vi "gfitsio-open-create-replace-file.vi"(4 "advisory dialog? (display:T)":bool=TRUE, 5 "prompt":string, 6 "default name":string, 8 "error in (no error)":errorcluster, 9 "function (open)":T2(ring), 11 "file path (dialog if empty)":path) -> (0 "error out":errorcluster, 2 "new file path":path, 3 "gfits refnum":T1)   [LabVIEW 2013, in "gfitsio.lvlib"]
doc: "Opens an existing FITS file, creates a new FITS file, or replaces an existing FITS file, programmatically or interactively using a file dialog box. You can optionally specify a dialog prompt and default file name."
uses:
  gfitsio.lvlib
  gfitsio-refnum.ctl
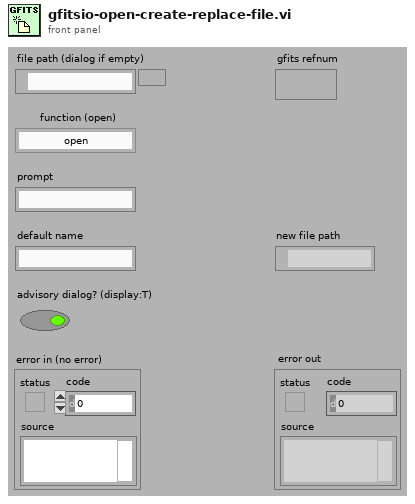
[diagram p1: front panel]
types:
  T1 = typedef "gfitsio.lvlib/gfitsio-refnum.ctl" = refnum<k1>
  T2 = enum16{"open", "open or create", "create or replace", "create", "open (read only)"}
  T3 = enum32{"existing file", "new file", "new or existing file", "existing dir", "new dir", "new or existing dir", "existing file (use LLBs)", "new file (use LLBs)", "new or existing file (use LLBs)", "new or existing file or directory (use LLBs)"}[]
  T4 = enum32{"existing file", "new file", "new or existing file", "existing dir", "new dir", "new or existing dir", "existing file (use LLBs)", "new file (use LLBs)", "new or existing file (use LLBs)", "new or existing file or directory (use LLBs)"}
  T5 = enum16{"Error", "Ok", "Cancel", "Abort", "Retry", "Ignore", "Yes", "No", "Close", "Help", "Disabled"}
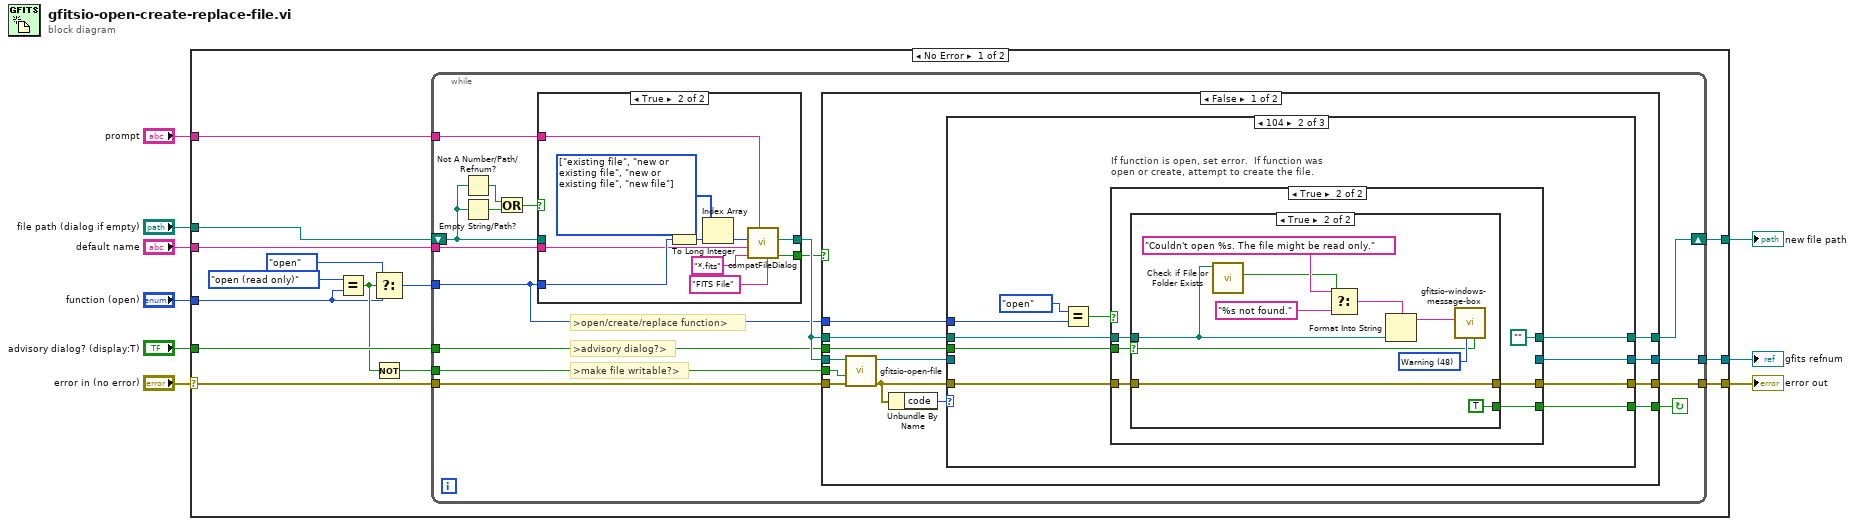
[diagram p0: block diagram]
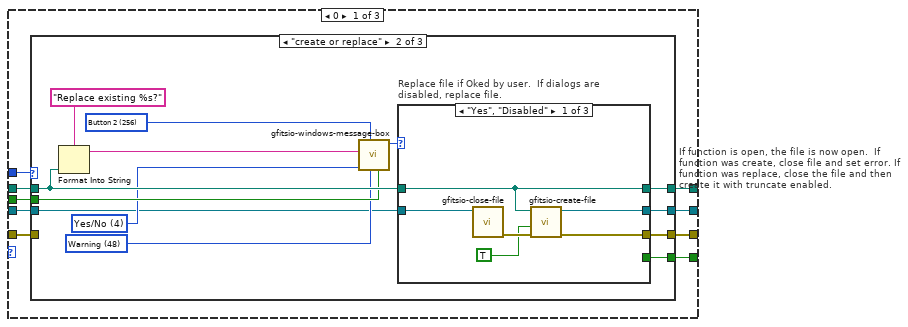
[diagram p3: hidden frame]
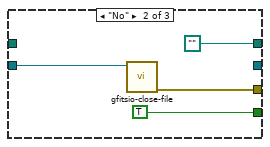
[diagram p5: hidden frame]
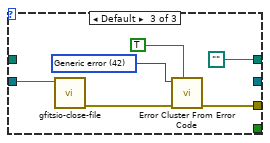
[diagram p6: hidden frame]
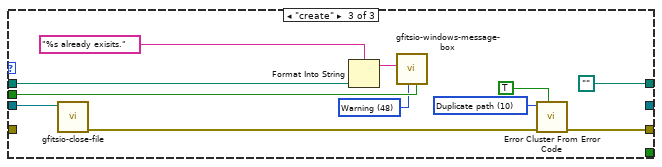
[diagram p7: hidden frame]
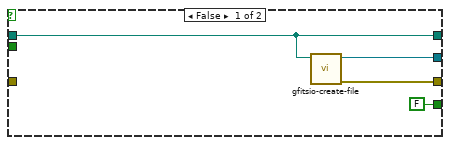
[diagram p8: hidden frame]
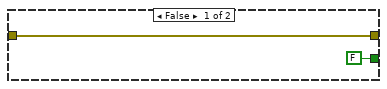
[diagram p9: hidden frame]
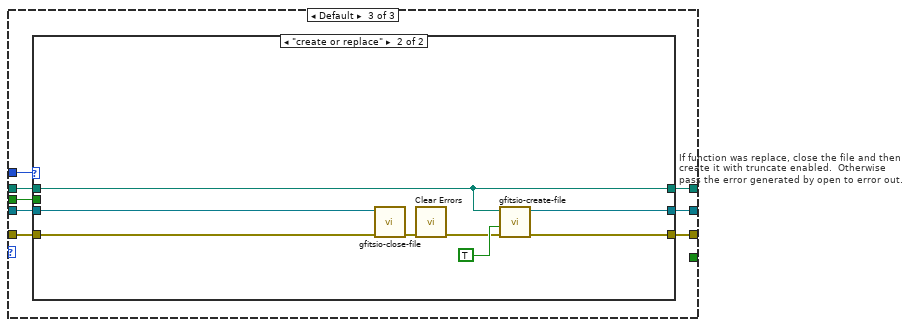
[diagram p10: hidden frame]
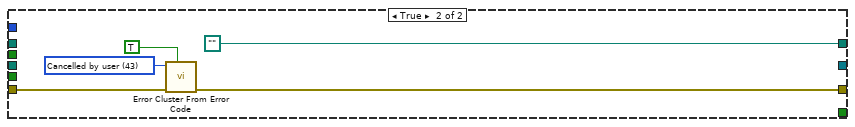
[diagram p12: hidden frame]
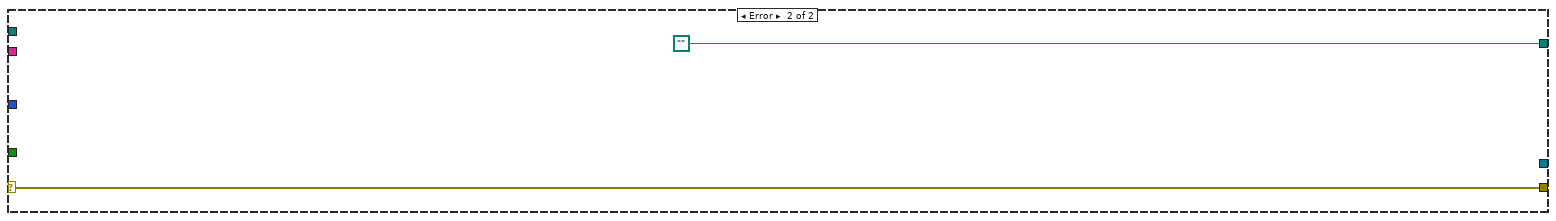
[diagram p13: hidden frame]
diagram:
  n1 = case shown="No Error" "error in (no error)" {
    selector: "error in (no error)" -> [w20 w172]
    tunnel: [w23 w172] -> w9
    tunnel: "advisory dialog? (display:T)" -> [w22 _]
    tunnel: [w21 path ""] -> w8
    tunnel: "default name" -> [w19 _]
    tunnel: "file path (dialog if empty)" -> [w18 _]
    tunnel: "prompt" -> [w17 _]
    tunnel: [w16 _] -> w3
    tunnel: "function (open)" -> [w11 _]
    frame No Error {
      n2 = Equal?(x=T2."open (read only)" ("y"), y=w11) -> (x = y?=w15:bool)
      n3 = Select(t=T2."open", s=w15, f=w11) -> (s? t:f=w12:T2)
      n4 = Not(x=w15) -> (.not. x?=w10:bool)
      n5 = while {
        tunnel: [w39] -> w23
        tunnel: w22 -> [w34]
        tunnel: w20 -> [w32]
        tunnel: w12 -> [w31]
        tunnel: w19 -> [w29]
        tunnel: w17 -> [w27]
        tunnel: w10 -> [w25]
        tunnel: [w24] -> w16
        shift-right: [w33] -> w21
        shift-left: w18 -> [w28]
        stop <- w26 continue-if-true
        # ">open/create/replace function>"
        # ">make file writable?>"
        # ">advisory dialog?>"
        n6 = Not A Number/Path/Refnum?(number/path/refnum=w28) -> (NaN/Path/Refnum?=w37:bool)
        n7 = Empty String/Path?(string/path=w28) -> (empty?=w36:bool)
        n8 = Or(x=w37, y=w36) -> (x .or. y?=w38:bool)
        n9 = case shown="True" w38 {
          tunnel: [_ w50] -> w30
          tunnel: [w40 w49] -> w35
          tunnel: w31 -> [_ w48]
          tunnel: w27 -> [_ w45]
          tunnel: w29 -> [_ w44]
          tunnel: w28 -> [w40 _]
          frame False {
            # "a File Path is supplied (not empty); proceed"
          }
          frame True {
            w46 = T3 [enum."existing file", enum."new or existing file", enum."new or existing file", enum."new file"] items=["existing file", "new file", "new or existing file", "existing dir", "new dir", "new or existing dir", "existing file (use LLBs)", "new file (use LLBs)", "new or existing file (use LLBs)", "new or existing file or directory (use LLBs)"]
            n10 = To Long Integer(number=w48) -> (32bit integer=w41:i32)
            n11 = Index Array(array=w46, index=w41) -> (element=w47:T4)
            n12 = call <vilib>:"compatFileDialog.vi"("pattern label"="FITS File", "prompt"=w45, "pattern"="*.fits", "default name"=w44, "select mode (2)"=w47) -> ("cancelled"=w50:bool, "path"=w49:path)  [unwired: 2 in, 3 out]
          }
        }
        n13 = case shown="False" w30 {
          tunnel: w31 -> [w63 _]
          tunnel: w32 -> [w62 w169]
          tunnel: [w58 w168] -> w39
          tunnel: w35 -> [w61 _]
          tunnel: w35 -> [w60 _]
          tunnel: w34 -> [w59 _]
          tunnel: [w57 path ""] -> w33
          tunnel: [w54 _] -> w26
          tunnel: w25 -> [w53 _]
          tunnel: [w51 _] -> w24
          frame False {
            n14 = call "gfitsio-open-file.vi"("error in (no error)"=w62, "read only? (T:no)"=w53, "path"=w61) -> ("error out"=w55:errorcluster, "gfits refnum"=w52:T1)  [unwired: 7 out]
            n15 = Unbundle By Name(w55) -> ("code"=w56:i32)
            n16 = case shown="104" w56 {
              tunnel: w63 -> [w72 w124 w155]
              tunnel: w60 -> [w70 w123 w153]
              tunnel: w59 -> [w71 w122 w154]
              tunnel: [w68 w121 w151] -> w58
              tunnel: [w69 w120 w152] -> w57
              tunnel: w55 -> [w67 w118 w150]
              tunnel: [w66 w116 _] -> w54
              tunnel: w52 -> [w65 _ w148]
              tunnel: [w64 w117 w149] -> w51
              frame 0 {
                n17 = case "If function is open, the file is now open.  If function was create, close file and set error. If function was replace, close the file and then create it with truncate enabled." shown="\"create or replace\"" w72 {
                  tunnel: w71 -> [_ w85 w114]
                  tunnel: w70 -> [w75 w86 w113]
                  tunnel: [w75 w88 path ""] -> w69
                  tunnel: w67 -> [w74 _ _]
                  tunnel: [w74 w87 w111] -> w68
                  tunnel: [_ w79 _] -> w66
                  tunnel: w65 -> [w73 w77 w105]
                  tunnel: [w73 w76 _] -> w64
                  frame "open", "open or create", "open (read only)" {
                  }
                  frame "create or replace" {
                    w80 = u32 256 items=["Button 1"=0, "Button 2"=256, "Button 3"=512, "Button 4"=1024] ("Default (Button 1)")
                    w81 = u32 4 items=["Abort/Retry/Ignore"=2, "OK"=0, "OK/Cancel"=1, "Retry/Cancel"=5, "Yes/No"=4, "Yes/No/Cancel"=3] ("Buttons (OK)")
                    w82 = u32 48 items=["None"=0, "Warning"=48, "Confirmation"=64, "Question"=32, "Error"=16, "User Icon"=128] ("Icon (None)")
                    n18 = Format Into String(format string="Replace existing %s?", w86) -> (resulting string=w78:string)  [unwired: 2 in, 1 out]
                    n19 = call "gfitsio-windows-message-box.vi"("enable dialog?"=w85, "Icon (None)"=w82, "Default (Button 1)"=w80, "Buttons (OK)"=w81, "Text"=w78) -> ("Button Selected"=w83:T5)  [unwired: 3 in, 3 out]
                    n20 = case "Replace file if Oked by user.  If dialogs are disabled, replace file." shown="\"Yes\", \"Disabled\"" w83 {
                      tunnel: [w92 path "" path ""] -> w88
                      tunnel: [w93 w97 w102] -> w87
                      tunnel: w86 -> [w92 _ _]
                      tunnel: [_ TRUE _] -> w79
                      tunnel: w77 -> [w90 w95 w99]
                      tunnel: [w89 _ _] -> w76
                      frame "Yes", "Disabled" {
                        n21 = call "gfitsio-close-file.vi"("gfits refnum"=w90) -> ("error out"=w94:errorcluster)  [unwired: 1 in, 9 out]
                        n22 = call "gfitsio-create-file.vi"("error in (no error)"=w94, "overwrite? (F:no)"=TRUE ("overwrite (F)"), "path"=w92) -> ("error out"=w93:errorcluster, "gfits refnum"=w89:T1)  [unwired: 7 out]
                      }
                      frame "No" {
                        n23 = call "gfitsio-close-file.vi"("gfits refnum"=w95) -> ("error out"=w97:errorcluster)  [unwired: 1 in, 9 out]
                      }
                      frame Default {
                        w101 = 42 items=["No error", "Argument error", "Memory is full", "Out of zone", "End of file", "File already open", "Generic file I/O error", "File not found", "File permission error", "Disk is full", "Duplicate path", "Too many files open", "System feature not enabled", "Resource file not found", "Cannot add resource", "Resource not found", "Image not found", "Image memory error", "Pen does not exist", "Config type invalid", "Config token not found", "Config parse error", "Config memory error", "Bad external code format", "Bad external code offset", "External code not present", "Null window", "Destroy window error", "Null menu", "Print aborted", "Bad print record", "Print driver error", "Windows error during printing", "Memory error during printing", "Print dialog error", "Generic print error", "Invalid device refnum", "Device not found", "Device parameter error", "Device unit error", "Cannot open device", "Device call aborted", "Generic error", "Cancelled by user", "Object ID too low", "Object ID too high", "Object not in heap", "Unknown heap", "Unknown object (invalid DefProc)", "Unknown object (DefProc not in table)", "Message out of range", "Invalid (null) method", "Unknown message", "Manager call not supported", "Bad address", "Network operation in progress", "Network operation timed out", "Connection is busy", "Network attribute not supported", "Network error", "Address in use", "System out of memory", "Connection aborted", "Connection refused", "Not connected", "Already connected", "Connection closed", "Initialization error (interapplication manager)", "Bad occurrence", "Wait on unbound occurrence handler", "Occurrence queue overflow", "Datalog type conflict", "Unused", "Unrecognized type (interapplication manager)", "Memory corrupt", "Failed to make temporary DLL", "Old CIN version", "Drag socket not found", "Failed to load drop-object", "Failed to register OLE object", "Failed to release OLE object", "Format specifier type mismatch", "Unknown format specifier", "Too few format specifiers", "Too many format specifiers", "Scan failed", "Newer CIN version", "Error converting to variant", "Runtime menu error", "Password tampered", "Variant attribute not found", "Incompatible variant data type", "Event data is not available", "Event Store is not present", "Occurrence is not found", "Event Queue is not created", "Event info is not available in the type library", "Refnum passed is NULL", "Error retrieving Class GUID", "Error retrieving CoClass GUID", "Error retrieving TypeLib GUID.", "Bad built application magic bytes.", "Specific driver is different from the specific driver associated with the Logical Name.", "There is no session opened to the class driver.", "Max Error", "MAX - Error with config objects", "MAX - Error loading configuration", "MAX - Group not supported", "Singlecast connections can not send to multicast addresses.", "Multicast connections can not send to singlecast addresses.", "Specified IP address not in multicast address range.", "Attempt to write to read-only multicast connection.", "Attempt to read from write-only multicast connection.", "The buffer used to receive a datagram was smaller than the datagram itself"]
                        n24 = call "gfitsio-close-file.vi"("gfits refnum"=w99) -> ("error out"=w103:errorcluster)  [unwired: 1 in, 9 out]
                        n25 = call <vilib>:"Error Cluster From Error Code.vi"("show call chain? (False)"=TRUE, "error in (no error)"=w103, "error code (0)"=w101) -> ("error out"=w102:errorcluster)  [unwired: 6 out]
                      }
                    }
                  }
                  frame "create" {
                    w106 = u32 48 items=["None"=0, "Warning"=48, "Confirmation"=64, "Question"=32, "Error"=16, "User Icon"=128] ("Icon (None)")
                    w109 = 10 items=["No error", "Argument error", "Memory is full", "Out of zone", "End of file", "File already open", "Generic file I/O error", "File not found", "File permission error", "Disk is full", "Duplicate path", "Too many files open", "System feature not enabled", "Resource file not found", "Cannot add resource", "Resource not found", "Image not found", "Image memory error", "Pen does not exist", "Config type invalid", "Config token not found", "Config parse error", "Config memory error", "Bad external code format", "Bad external code offset", "External code not present", "Null window", "Destroy window error", "Null menu", "Print aborted", "Bad print record", "Print driver error", "Windows error during printing", "Memory error during printing", "Print dialog error", "Generic print error", "Invalid device refnum", "Device not found", "Device parameter error", "Device unit error", "Cannot open device", "Device call aborted", "Generic error", "Cancelled by user", "Object ID too low", "Object ID too high", "Object not in heap", "Unknown heap", "Unknown object (invalid DefProc)", "Unknown object (DefProc not in table)", "Message out of range", "Invalid (null) method", "Unknown message", "Manager call not supported", "Bad address", "Network operation in progress", "Network operation timed out", "Connection is busy", "Network attribute not supported", "Network error", "Address in use", "System out of memory", "Connection aborted", "Connection refused", "Not connected", "Already connected", "Connection closed", "Initialization error (interapplication manager)", "Bad occurrence", "Wait on unbound occurrence handler", "Occurrence queue overflow", "Datalog type conflict", "Unused", "Unrecognized type (interapplication manager)", "Memory corrupt", "Failed to make temporary DLL", "Old CIN version", "Drag socket not found", "Failed to load drop-object", "Failed to register OLE object", "Failed to release OLE object", "Format specifier type mismatch", "Unknown format specifier", "Too few format specifiers", "Too many format specifiers", "Scan failed", "Newer CIN version", "Error converting to variant", "Runtime menu error", "Password tampered", "Variant attribute not found", "Incompatible variant data type", "Event data is not available", "Event Store is not present", "Occurrence is not found", "Event Queue is not created", "Event info is not available in the type library", "Refnum passed is NULL", "Error retrieving Class GUID", "Error retrieving CoClass GUID", "Error retrieving TypeLib GUID.", "Bad built application magic bytes.", "Specific driver is different from the specific driver associated with the Logical Name.", "There is no session opened to the class driver.", "Max Error", "MAX - Error with config objects", "MAX - Error loading configuration", "MAX - Group not supported", "Singlecast connections can not send to multicast addresses.", "Multicast connections can not send to singlecast addresses.", "Specified IP address not in multicast address range.", "Attempt to write to read-only multicast connection.", "Attempt to read from write-only multicast connection.", "The buffer used to receive a datagram was smaller than the datagram itself"]
                    n26 = call "gfitsio-close-file.vi"("gfits refnum"=w105) -> ("error out"=w110:errorcluster)  [unwired: 1 in, 9 out]
                    n27 = Format Into String(format string="%s already exisits.", w113) -> (resulting string=w107:string)  [unwired: 2 in, 1 out]
                    n28 = call "gfitsio-windows-message-box.vi"("enable dialog?"=w114, "Icon (None)"=w106, "Text"=w107) -> ()  [unwired: 4 in, 5 out]
                    n29 = call <vilib>:"Error Cluster From Error Code.vi"("show call chain? (False)"=TRUE, "error in (no error)"=w110, "error code (0)"=w109) -> ("error out"=w111:errorcluster)  [unwired: 6 out]
                  }
                }
              }
              frame 104 {
                n30 = Equal?(x=T2."open", y=w124) -> (x = y?=w125:bool)
                n31 = case "If function is open, set error.  If function was open or create, attempt to create the file." shown="True" w125 {
                  tunnel: [w128 path ""] -> w120
                  tunnel: w123 -> [w128 w134]
                  tunnel: w122 -> [_ w131]
                  tunnel: w118 -> [_ w133]
                  tunnel: [w129 w132] -> w121
                  tunnel: [w127 _] -> w117
                  tunnel: [FALSE w130] -> w116
                  frame False {
                    n32 = call "gfitsio-create-file.vi"("path"=w128) -> ("error out"=w129:errorcluster, "gfits refnum"=w127:T1)  [unwired: 2 in, 7 out]
                  }
                  frame True {
                    n33 = case shown="True" w131 {
                      selector: w131 -> [_ w139]
                      tunnel: w134 -> [_ w145]
                      tunnel: w133 -> [w137 w140]
                      tunnel: [w137 w140] -> w132
                      tunnel: [FALSE TRUE] -> w130
                      frame False {
                      }
                      frame True {
                        w146 = u32 48 items=["None"=0, "Warning"=48, "Confirmation"=64, "Question"=32, "Error"=16, "User Icon"=128] ("Icon (None)")
                        n34 = call <vilib>:"Check if File or Folder Exists.vi"("path"=w145) -> ("file or folder exists?"=w143:bool)  [unwired: 8 in, 2 out]
                        n35 = Select(t="Couldn't open %s. The file might be read only." ("format string"), s=w143, f="%s not found." ("format string")) -> (s? t:f=w141:string)
                        n36 = Format Into String(format string=w141, w145) -> (resulting string=w147:string)  [unwired: 2 in, 1 out]
                        n37 = call "gfitsio-windows-message-box.vi"("enable dialog?"=w139, "Icon (None)"=w146, "Text"=w147) -> ()  [unwired: 4 in, 5 out]
                      }
                    }
                  }
                }
              }
              frame Default {
                n38 = case "If function was replace, close the file and then create it with truncate enabled.  Otherwise pass the error generated by open to error out." shown="\"create or replace\"" w155 {
                  tunnel: w154 -> [_ _]
                  tunnel: w153 -> [w158 w165]
                  tunnel: [w158 w165] -> w152
                  tunnel: w150 -> [w157 w166]
                  tunnel: [w157 w164] -> w151
                  tunnel: [w156 w160] -> w149
                  tunnel: w148 -> [w156 w159]
                  frame "open", "open or create", "create", "open (read only)" {
                  }
                  frame "create or replace" {
                    n39 = call "gfitsio-close-file.vi"("error in (no error)"=w166, "gfits refnum"=w159) -> ("error out"=w162:errorcluster)  [unwired: 9 out]
                    n40 = call <vilib>:"Clear Errors.vi"("error in (no error)"=w162) -> ("error out"=w161:errorcluster)  [unwired: 6 out]
                    n41 = call "gfitsio-create-file.vi"("error in (no error)"=w161, "overwrite? (F:no)"=TRUE ("overwrite (F)"), "path"=w165) -> ("error out"=w164:errorcluster, "gfits refnum"=w160:T1)  [unwired: 7 out]
                  }
                }
              }
            }
          }
          frame True {
            w171 = 43 items=["No error", "Argument error", "Memory is full", "Out of zone", "End of file", "File already open", "Generic file I/O error", "File not found", "File permission error", "Disk is full", "Duplicate path", "Too many files open", "System feature not enabled", "Resource file not found", "Cannot add resource", "Resource not found", "Image not found", "Image memory error", "Pen does not exist", "Config type invalid", "Config token not found", "Config parse error", "Config memory error", "Bad external code format", "Bad external code offset", "External code not present", "Null window", "Destroy window error", "Null menu", "Print aborted", "Bad print record", "Print driver error", "Windows error during printing", "Memory error during printing", "Print dialog error", "Generic print error", "Invalid device refnum", "Device not found", "Device parameter error", "Device unit error", "Cannot open device", "Device call aborted", "Generic error", "Cancelled by user", "Object ID too low", "Object ID too high", "Object not in heap", "Unknown heap", "Unknown object (invalid DefProc)", "Unknown object (DefProc not in table)", "Message out of range", "Invalid (null) method", "Unknown message", "Manager call not supported", "Bad address", "Network operation in progress", "Network operation timed out", "Connection is busy", "Network attribute not supported", "Network error", "Address in use", "System out of memory", "Connection aborted", "Connection refused", "Not connected", "Already connected", "Connection closed", "Initialization error (interapplication manager)", "Bad occurrence", "Wait on unbound occurrence handler", "Occurrence queue overflow", "Datalog type conflict", "Unused", "Unrecognized type (interapplication manager)", "Memory corrupt", "Failed to make temporary DLL", "Old CIN version", "Drag socket not found", "Failed to load drop-object", "Failed to register OLE object", "Failed to release OLE object", "Format specifier type mismatch", "Unknown format specifier", "Too few format specifiers", "Too many format specifiers", "Scan failed", "Newer CIN version", "Error converting to variant", "Runtime menu error", "Password tampered", "Variant attribute not found", "Incompatible variant data type", "Event data is not available", "Event Store is not present", "Occurrence is not found", "Event Queue is not created", "Event info is not available in the type library", "Refnum passed is NULL", "Error retrieving Class GUID", "Error retrieving CoClass GUID", "Error retrieving TypeLib GUID.", "Bad built application magic bytes.", "Specific driver is different from the specific driver associated with the Logical Name.", "There is no session opened to the class driver.", "Max Error", "MAX - Error with config objects", "MAX - Error loading configuration", "MAX - Group not supported", "Singlecast connections can not send to multicast addresses.", "Multicast connections can not send to singlecast addresses.", "Specified IP address not in multicast address range.", "Attempt to write to read-only multicast connection.", "Attempt to read from write-only multicast connection.", "The buffer used to receive a datagram was smaller than the datagram itself"]
            n42 = call <vilib>:"Error Cluster From Error Code.vi"("show call chain? (False)"=TRUE, "error in (no error)"=w169, "error code (0)"=w171) -> ("error out"=w168:errorcluster)  [unwired: 6 out]
          }
        }
      }
    }
    frame Error {
    }
  }
  "new file path" <- w8
  "error out" <- w9
  "gfits refnum" <- w3
